vi "Target Distance.vi"   [LabVIEW 2019]
uses:
  <vilib>/Rock Robotics/Network Tables/NT Read Number.vi
  Robot Global Data.vi
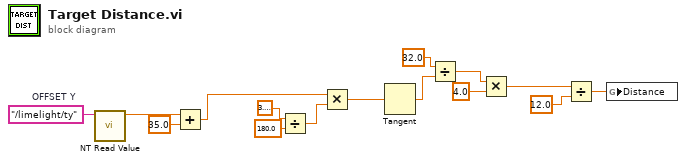
[diagram p0: block diagram]
diagram:
  w7 = "/limelight/ty"  # OFFSET Y
  n1 = call-poly <vilib>:"NT Read Value.vi"("Name"=w7) -> ("Numeric"=w9:dbl)  [unwired: 9 in, 1 out]
  n2 = Add(x=w9, y=35.0) -> (x+y=w11:dbl)
  n3 = Divide(x=3.141592653589793, y=180.0) -> (x/y=w2:dbl)
  n4 = Multiply(x=w11, y=w2) -> (x*y=w3:dbl)
  n5 = Tangent(1:w3) -> (0:w4:dbl)
  n6 = Divide(x=32.0, y=w4) -> (x/y=w12:dbl)
  n7 = Multiply(x=w12, y=4.0) -> (x*y=w15:dbl)
  n8 = Divide(x=w15, y=12.0) -> (x/y=w1:dbl)
  n9 = global write "Robot Global Data.vi" "Distance"(w1) -> ()
